vi "provide_OME_data.vi"(6 "image ID":string, 8 "error in (no error)":errorcluster, 9 "structuredAttribute string in":string, 10 "OME element in":refnum<class "XMLElement.lvclass">, 11 "GenericPlugin in":refnum<class "GenericComponent.lvclass">) -> (0 "error out":errorcluster, 1 "structuredAttribute string out":string, 2 "OME element out":refnum<class "XMLElement.lvclass">, 3 "GenericPlugin out":refnum<class "GenericComponent.lvclass">)   [LabVIEW 2010, in "GenericComponent.lvclass"]
uses:
  GenericComponent.lvclass
  XMLElement/XMLElement/XMLElement.lvclass
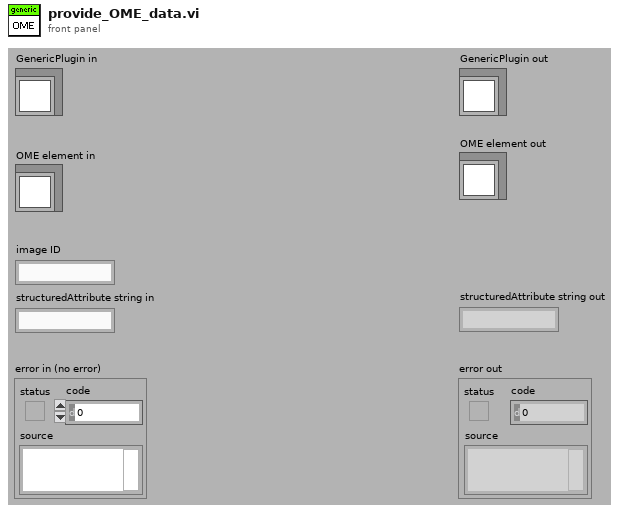
[diagram p1: front panel]
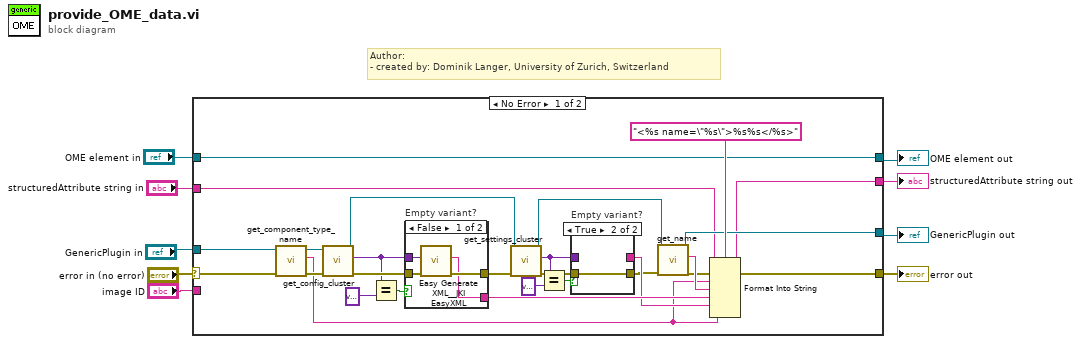
[diagram p0: block diagram]
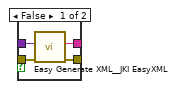
[diagram p2: hidden frame]
diagram:
  # "Author: \n- created by: Dominik Langer, University of Zurich, Switzerland"
  n1 = case shown="No Error" "error in (no error)" {
    selector: "error in (no error)" -> [w22 w50]
    tunnel: "GenericPlugin in" -> [w21 w49]
    tunnel: [w17 w50] -> w7
    tunnel: [w23 w49] -> w6
    tunnel: [w18 w48] -> w3
    tunnel: "OME element in" -> [w18 w48]
    tunnel: "image ID" -> [_ _]
    tunnel: "structuredAttribute string in" -> [w20 w47]
    tunnel: [w19 w47] -> w1
    frame No Error {
      n2 = call-dynamic "get_component_type_name.vi"("error in (no error)"=w22, "GenericPlugin in"=w21) -> ("error out"=w33:errorcluster, "component type"=w16:string, "GenericPlugin out"=w32:refnum<class "GenericComponent.lvclass">)  [unwired: 7 in]
      n3 = call-dynamic "get_config_cluster.vi"("error in (no error)"=w33, "GenericComponent in"=w32) -> ("error out"=w35:errorcluster, "config cluster (variant)"=w15:variant, "GenericComponent out"=w36:refnum<class "GenericComponent.lvclass">)  [unwired: 7 in]
      n4 = Equal?(x=w15, y=variant ("config cluster (variant)")) -> (x = y?=w13:bool)
      n5 = case "Empty variant?" shown="False" w13 {
        tunnel: w15 -> [w45 _]
        tunnel: w35 -> [w44 w46]
        tunnel: [w43 w46] -> w34
        tunnel: [w42 _] -> w31
        frame False {
          n6 = call <vilib>:"Easy Generate XML__JKI EasyXML.vi"("error in (no error)"=w44, "LabVIEW Data"=w45) -> ("error out"=w43:errorcluster, "XML String"=w42:string)  [unwired: 8 in]
        }
        frame True {
        }
      }
      n7 = call-dynamic "get_settings_cluster.vi"("error in (no error)"=w34, "GenericPlugin in"=w36) -> ("error out"=w30:errorcluster, "settings cluster"=w12:variant, "GenericPlugin out"=w24:refnum<class "GenericComponent.lvclass">)  [unwired: 7 in]
      n8 = Equal?(x=w12, y=variant ("config cluster (variant)")) -> (x = y?=w10:bool)
      n9 = case "Empty variant?" shown="True" w10 {
        tunnel: w30 -> [w40 w41]
        tunnel: w12 -> [w39 _]
        tunnel: [w38 _] -> w29
        tunnel: [w37 w41] -> w26
        frame False {
          n10 = call <vilib>:"Easy Generate XML__JKI EasyXML.vi"("error in (no error)"=w40, "LabVIEW Data"=w39) -> ("error out"=w37:errorcluster, "XML String"=w38:string)  [unwired: 8 in]
        }
        frame True {
        }
      }
      n11 = call-dynamic "get_name.vi"("error in (no error)"=w26, "GenericPlugin in"=w24) -> ("error out"=w25:errorcluster, "component name"=w28:string, "GenericPlugin out"=w23:refnum<class "GenericComponent.lvclass">)  [unwired: 7 in]
      n12 = Format Into String(format string="<%s name=\"%s\">%s%s</%s>", initial string=w20, error in=w25, w16, w28, w31, w29, w16) -> (resulting string=w19:string, error out=w17:errorcluster)
    }
    frame Error {
    }
  }
  "error out" <- w7
  "GenericPlugin out" <- w6
  "OME element out" <- w3
  "structuredAttribute string out" <- w1
